vi "Mask Write Holding Register.vi"(4 "OR Mask":u16, 6 "AND Mask":u16, 7 "unit ID":u8, 8 "error in":errorcluster, 10 "address":u16, 11 "Modbus instance in":refnum<class "Modbus Slave.lvclass">) -> (0 "error out":errorcluster, 3 "Modbus instance out":refnum<class "Modbus Slave.lvclass">)   [LabVIEW 2013, in "Modbus Library - Advance.lvlib" / "Modbus Slave.lvclass"]
doc: "Writes the masked value of a single register using an <b>AND mask</b> and an <b>OR mask</b> using the equation below:\nResult=(Current Value AND AndMask) OR (OrMask AND !AndMask)"
uses:
  Modbus Slave.lvclass
  Modbus Slave.lvclass/Modbus Slave.ctl
  Standard Data Model/Standard Data Model.lvclass
  Super Data Model/Super Data Model.lvclass
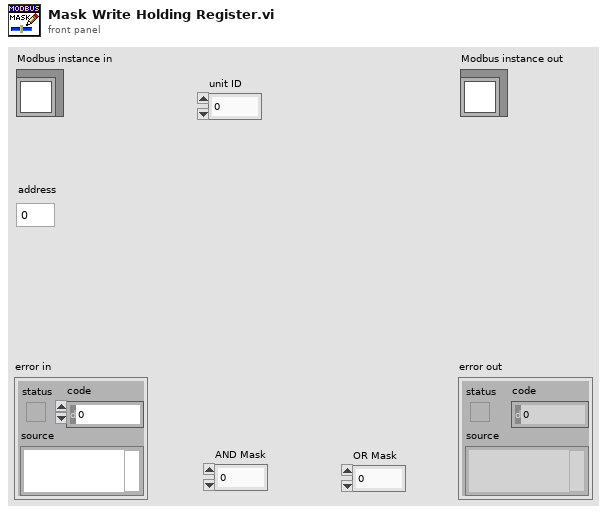
[diagram p1: front panel]
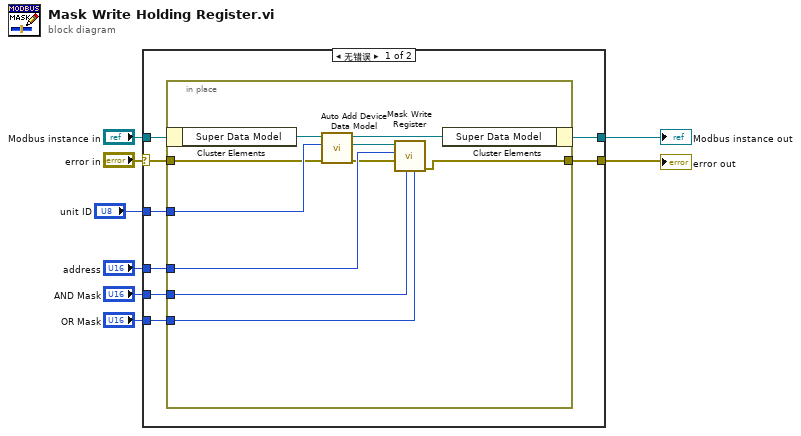
[diagram p0: block diagram]
diagram:
  n1 = case shown="无错误" "error in" {
    selector: "error in" -> [w14 w28]
    tunnel: [w15 w28] -> w7
    tunnel: "Modbus instance in" -> [w16 w27]
    tunnel: [w13 w27] -> w8
    tunnel: "address" -> [w12 _]
    tunnel: "AND Mask" -> [w11 _]
    tunnel: "OR Mask" -> [w10 _]
    tunnel: "unit ID" -> [w9 _]
    frame No Error {
      n2 = in-place {
        in-place-border: [w26] -> w15
        in-place-border: w14 -> [w20]
        in-place-border: w12 -> [w25]
        in-place-border: w11 -> [w24]
        in-place-border: w10 -> [w23]
        in-place-border: w9 -> [w21]
        n3 = in-place-cluster #1(w16) -> ("Super Data Model"=w22:refnum<class "Super Data Model.lvclass">)
        n4 = call "Auto Add Device Data Model.vi"("error in"=w20, "unit ID"=w21, "Super Data Model in"=w22) -> ("error out"=w18:errorcluster, "device data model"=w19:refnum<class "Standard Data Model.lvclass">, "Super Data Model out"=w17:refnum<class "Super Data Model.lvclass">)  [unwired: 6 in]
        n5 = call-dynamic "Mask Write Register.vi"("OR Mask"=w23, "AND Mask"=w24, "error in"=w18, "address"=w25, "device data model in"=w19) -> ("error out"=w26:errorcluster)  [unwired: 5 in, 1 out]
        n6 = in-place-cluster #1("Super Data Model"=w17) -> (w13:refnum<class "Modbus Slave.lvclass">)
      }
    }
    frame Error {
    }
  }
  "error out" <- w7
  "Modbus instance out" <- w8
